vi "Error Queue Reference.vi"() -> ()   [LabVIEW 2018]
panel:
  out "Queue Errores":refnum<queue>
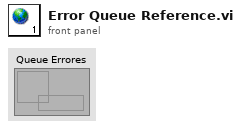
[diagram p1: front panel]
diagram:
